vi "Test RD Retrieval - Target.vi"() -> ()   [LabVIEW 2015]
uses:
  <vilib>/FPGAPlugInAG/cRIO-9081/niLvFpga_Open_cRIO-9081.vi
  <vilib>/Utility/error.llb/Error Cluster From Error Code.vi
  <vilib>/rvi/errors/niLvFpgaAdjustHostInterfaceError.vi
  <vilib>/rvi/interface/common/niFpgaWaitOnOcc.vi
  <vilib>/RVI Host/nirviSupport.llb/nirviErrorClusterFromErrorCode.vi
  <vilib>/FPGAPlugInAG/cRIO-9081/niLvFpga_Close_cRIO-9081.vi
  <vilib>/rvi/interface/nirviOpenFPGA/nirviOpenFPGA.xnode
  FPGA Bitfiles/Nicholas_FPGATarget_TestRD_yTEjeKL8TuA.lvbitx
  <vilib>/rvi/interface/nirviReadWriteControl/nirviReadWriteControl.xnode
  <vilib>/rvi/interface/nirviMethod/nirviMethod.xnode
  <vilib>/rvi/interface/nirviCloseFPGA/nirviCloseFPGA.xnode
  <vilib>/rvi/errors/niLvFpgaMergeErrorWithErrorCode.vi
  NiFpgaLv.dll
  <vilib>/FPGAPlugInAG/cRIO-9081/niLvFpga_ConfigureFifo_cRIO-9081.vi
  <vilib>/FPGAPlugInAG/cRIO-9081/niLvFpga_StartFifo_cRIO-9081.vi
  <vilib>/FPGAPlugInAG/cRIO-9081/niLvFpga_ReadFifo_cRIO-9081.vi
  <vilib>/rvi/interface/nirviMethod/StockFPGA_InlinedMethodWaitForSingleIRQ.vi
  <vilib>/FPGAPlugInAG/cRIO-9081/niLvFpga_WaitOnIrq_cRIO-9081.vi
  <vilib>/FPGAPlugInAG/cRIO-9081/niLvFpga_AcknowledgeIrq_cRIO-9081.vi
panel:
  out "Waveform Graph 3":i16[](graph)
  in  "Num2Acq":u16=500
  out "Waveform Graph 2":sgl[][](graph)
  out "Waveform Chart":cluster{i32, sgl}(graph)={388, 4622.0}
  in  "TotNumSamp":u16=1000
  in  "DC":u16=500
  out "error out 2":errorcluster
  out "error out":errorcluster
  out "x-y":dbl=2.071805000305176
  out "channel 0":sgl[](array[numeric])
  in  "Stop":bool
  out "Elements Remaining":u32=2903286
  in  "Number of Elements":u32=999870
  out "Actual Depth":u32=5000000
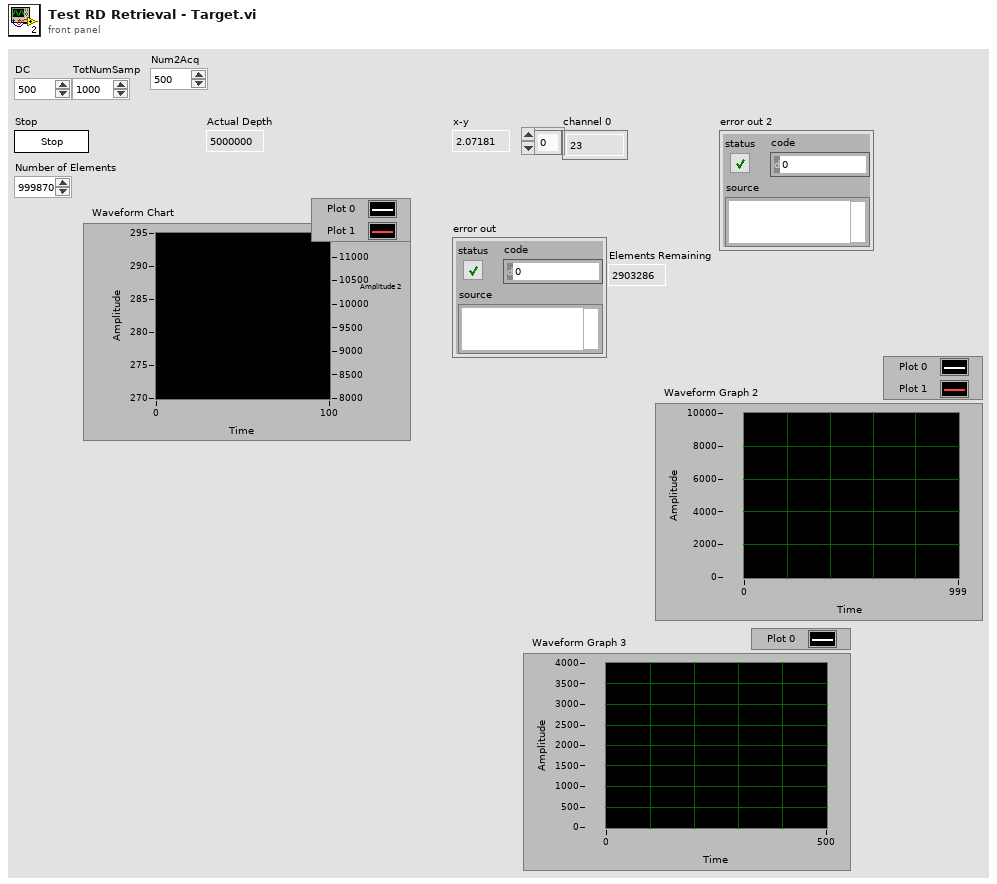
[diagram p1: front panel]
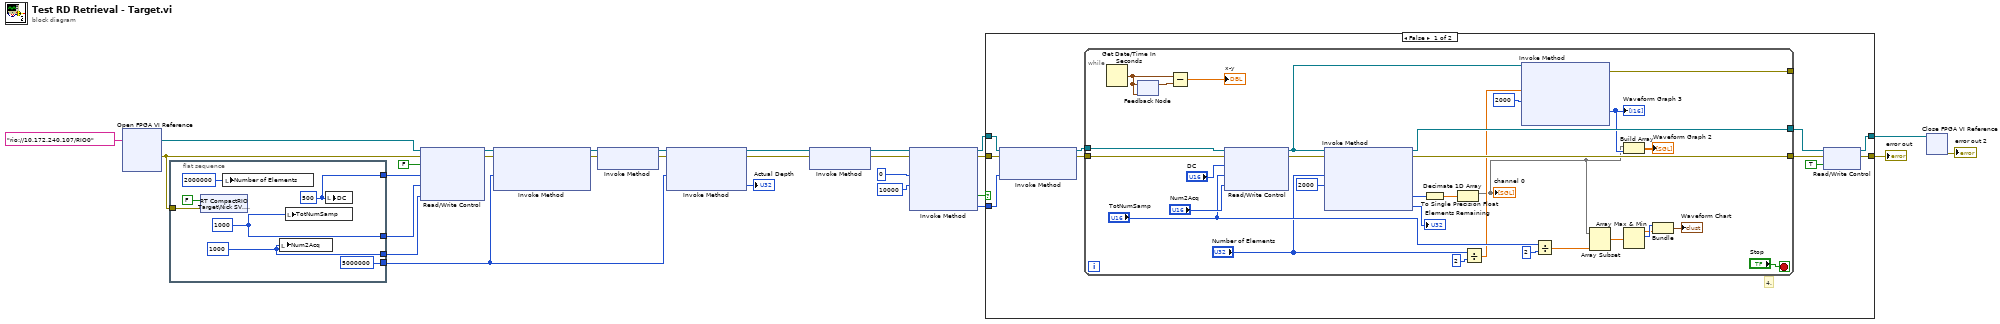
[diagram p0: block diagram]
diagram:
  n1 = xnode "Open FPGA VI Reference"("resource name"=tag "rio://10.172.240.107/RIO0") -> ("FPGA VI Reference Out"=w19:refnum<k20>, "error out"=w17:errorcluster)  [unwired: 1 in]
  n2 = flat-sequence {
    tunnel: w17 -> [w34]
    tunnel: [w33] -> w10
    tunnel: [w32] -> w9
    tunnel: [u32 5000000 ("Requested Depth")] -> w8
    tunnel: [w30] -> w1
    frame #0 {
      w30 = u16 1000 ("Num2Acq")
      w33 = u16 1000 ("TotNumSamp")
      w32 = u16 500 ("DC")
      n3 = shared-variable "RT CompactRIO Target\\Nick SV.lvlib\\Stop"(FALSE ("Stop"), error in=w34) -> ()  [unwired: 1 out]
      n4 = local write "Number of Elements"(u32 2000000 ("Number of Elements")) -> ()
      n5 = local write "Num2Acq"(w30) -> ()
      n6 = local write "TotNumSamp"(w33) -> ()
      n7 = local write "DC"(w32) -> ()
    }
  }
  n8 = xnode "Read/Write Control"("FPGA VI Reference In"=w19, "error in"=w17, "Stop"=FALSE, "DC"=w9, "TotNumSamp"=w10, "Num2Acq"=w1) -> ("FPGA VI Reference Out"=w7:refnum<k20>, "error out"=w4:errorcluster)
  n9 = xnode "Invoke Method"("FPGA VI Reference In"=w7, "error in"=w4, "Requested Depth"=w8) -> ("FPGA VI Reference Out"=w6:refnum<k20>, "error out"=w5:errorcluster)  [unwired: 1 out]
  n10 = xnode "Invoke Method"("FPGA VI Reference In"=w6, "error in"=w5) -> ("FPGA VI Reference Out"=w3:refnum<k20>, "error out"=w2:errorcluster)
  n11 = xnode "Invoke Method"("FPGA VI Reference In"=w3, "error in"=w2, "Requested Depth"=w8) -> ("FPGA VI Reference Out"=w12:refnum<k20>, "error out"=w11:errorcluster, "Actual Depth"=→"Actual Depth":u32)
  n12 = xnode "Invoke Method"("FPGA VI Reference In"=w12, "error in"=w11) -> ("FPGA VI Reference Out"=w20:refnum<k20>, "error out"=w18:errorcluster)
  n13 = xnode "Invoke Method"("FPGA VI Reference In"=w20, "error in"=w18, "IRQ Number(s)"=0, "Timeout (ms)"=10000) -> ("FPGA VI Reference Out"=w26:refnum<k20>, "error out"=w27:errorcluster, "Timed Out"=w15:bool, "IRQ(s) Asserted"=w25:i32)
  n14 = case shown="False" w15 {
    tunnel: w27 -> [w45 w78]
    tunnel: w26 -> [w44 w77]
    tunnel: w25 -> [w43 _]
    tunnel: [w40 w77] -> w22
    tunnel: [w36 w78] -> w14
    frame False {
      # "4."
      n15 = xnode "Invoke Method"("FPGA VI Reference In"=w44, "error in"=w45, "IRQ Number(s)"=w43) -> ("FPGA VI Reference Out"=w42:refnum<k20>, "error out"=w38:errorcluster)
      n16 = while {
        tunnel: w42 -> [w61]
        tunnel: [w58] -> w41
        tunnel: w38 -> [w60]
        tunnel: [w57] -> w37
        tunnel: [w53] -> _
        stop <- "Stop" stop-if-true
        n17 = Get Date/Time In Seconds() -> (seconds since 1Jan1904=w73:timestamp)
        n18 = feedback-in #1(w73) -> ()
        n19 = feedback #1(w73) -> (w76:timestamp)
        n20 = Subtract(x=w73, y=w76) -> (x-y=→"x-y":dbl)
        n21 = xnode "Read/Write Control"("FPGA VI Reference In"=w61, "error in"=w60, "DC"="DC", "TotNumSamp"="TotNumSamp", "Num2Acq"="Num2Acq") -> ("FPGA VI Reference Out"=w54:refnum<k20>, "error out"=w59:errorcluster)
        n22 = xnode "Invoke Method"("FPGA VI Reference In"=w54, "error in"=w59, "Number of Elements"="Number of Elements", "Timeout (ms)"=2000) -> ("FPGA VI Reference Out"=w58:refnum<k20>, "error out"=w57:errorcluster, "Data"=w72:i16[], "Elements Remaining"=→"Elements Remaining":u32)
        n23 = To Single Precision Float(number=w72) -> (single precision float=w74:sgl[])
        n24 = Decimate 1D Array(w74) -> (w47:sgl[])  [unwired: 1 out]
        "channel 0" <- w47
        n25 = Divide(x="Number of Elements", y=u32 2) -> (x/y=w49:dbl)
        n26 = xnode "Invoke Method"("FPGA VI Reference In"=w54, "Number of Elements"=w49, "Timeout (ms)"=2000) -> ("error out"=w53:errorcluster, "Data"=w48:i16[])  [unwired: 1 in, 2 out]
        "Waveform Graph 3" <- w48
        n27 = Divide(x="TotNumSamp", y=u16 2) -> (x/y=w63:dbl)
        n28 = Array Subset(array=w47, length=w63) -> (w69:sgl[])  [unwired: 1 in]
        n29 = Build Array(w47, w48) -> (→"Waveform Graph 2":sgl[][])
        n30 = Array Max & Min(array=w69) -> (max value=w67:sgl, max index (indices)=w68:i32)  [unwired: 2 out]
        n31 = Bundle(w68, w67) -> (→"Waveform Chart":cluster{i32, sgl})  [unwired: 1 in]
      }
      n32 = xnode "Read/Write Control"("FPGA VI Reference In"=w41, "error in"=w37, "Stop"=TRUE) -> ("FPGA VI Reference Out"=w40:refnum<k20>, "error out"=w36:errorcluster)
    }
    frame True {
    }
  }
  "error out" <- w14
  n33 = xnode "Close FPGA VI Reference"("FPGA VI Reference In"=w22) -> ("error out"=→"error out 2":errorcluster)  [unwired: 1 in]
